vi "Wind_Turbine_Global.vi"() -> ()   [LabVIEW 2010]
panel:
  in  "Radius (mm)":dbl
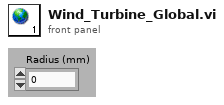
[diagram p1: front panel]
diagram:
